vi "setpoint_new(SubVI).vi"(0 "Filed 2":dbl=300.0, 1 "Field":dbl=300.0, 2 "type":T1, 3 "Rate/speed":dbl=10.0, 4 "Mode":i32(ring) items=["Persistent", "Driven"], 5 "输出簇 2":T2={"initialize"=enum."SR830", "6221"={"6221 Resource"="GPIB0::24::INSTR", "Delta status"=FALSE, "电流|RMS(A)"=0.0}, "SR830+6221"={"source"=0, "Current(A)"=0.0, "阻抗(Ohm)"=0.0, "SR830 1"=FALSE, "SR830 2"=FALSE, "SR830 3"=FALSE, "SR830 4"=FALSE, "VISA 1"="", "VISA 2"="", "VISA 3"="", "VISA 4"="", "Reserve 1"=0, "Reserve 2"=-1, "Reserve 3"=-1, "Reserve 4"=-1, "Sensitivity 1"=-1, "Sensitivity 2"=0, "Sensitivity 3"=-1, "Sensitivity 4"=-1, "量程入 1"=0, "量程入 2"=0, "量程入 3"=0, "量程入 4"=0}, "2400"={"2400"=FALSE, "VISA"="", "Output Level (0)"=1e-05, "Compliance  Level (0.1)"=10.0}, "ch"={"ch"=[], "current"=[], "change?"=[], "holding current\nwhen change ch?"=FALSE}, "Instrument"={"325 Resource "="GPIB0::24::INSTR", "Input (0:A) 325"=0, "Heater Output (1:1) 325"=1, "340 Resource"="GPIB0::24::INSTR", "Input (0:A) 340"=0, "Loop (0: 1)"=1, "Input (0:B) 340"=1, "Loop (1: 1)"=2, "340 Status"=refnum, "Instrument Type"=enum."PPMS-Rotate", "quantum design"=refnum, "semaphore 325"=refnum, "TCP master instance"=refnum, "M24C Resource"="GPIB0::24::INSTR", "4G supply"="GPIB0::24::INSTR", "Temp Status 24C"=refnum, "Temp"=refnum, "9T信号"=refnum, "limit"={"Field limit"=0.0, "Field rate limit"=0.0, "Temp limit"=0.0, "Temp low limit"=0.0, "Temp rate limit "=0.0}, "4g supply status"=refnum, "vi路径"="", "in-plane"="", "out-plane"="", "in-plane signal"=FALSE, "out-plane signal"=FALSE, "in plane 信号"=refnum, "pzt volt"=refnum, "Aborting"=refnum, "数据文件"=refnum, "warning"=refnum, "750 visa"="", "750 rotate"="", "335 Status 2"=refnum, "335 Resource "="GPIB0::24::INSTR", "Input (0:A) 335"=0, "Input (0:B) 335"=1, "Heater Output (1:1) 335"=1, "semaphore 340"=refnum, "semaphore 335"=refnum, "325 Status"=refnum, "semaphore 750"=refnum, "750 field status"=refnum}, "2614B"={"2614B chA"=FALSE, "2614B chB"=FALSE, "VISA"=""}, "33522b"={"33522b resource name"="", "零电压"=0.0, "最大电压"=148.0, "间隔"=4.0, "最小电压"=-48.0, "PZT Scan?"=FALSE}, "gating type"=enum."2614(daul)"} {"Instrument"."Loop (1: 1)" items=["1"=1, "2"=2]; "Instrument"."Loop (0: 1)" items=["1"=1, "2"=2]; "Instrument"."Input (0:B) 340" items=["A", "B", "C", "D"]; "Instrument"."Heater Output (1:1) 335" items=["1"=1, "2"=2]; "Instrument"."Input (0:B) 335" items=["A", "B"]; "Instrument"."Input (0:A) 335" items=["A", "B"]; "Instrument"."Heater Output (1:1) 325" items=["1"=1, "2"=2]; "Instrument"."Input (0:A) 325" items=["A", "B"]; "Instrument"."Input (0:A) 340" items=["1"=1, "2"=2]; "SR830+6221"."Sensitivity 4" items=["Auto Gain"=-1, "2 nV/fA"=0, "5 nV/fA"=1, "10 nV/fA"=2, "20 nV/fA"=3, "50 nV/fA"=4, "100 nV/fA"=5, "200 nV/fA"=6, "500 nV/fA"=7, "1 uV/pA"=8, "2 uV/pA"=9, "5 uV/pA"=10, "10 uV/pA"=11, "20 uV/pA"=12, "50 uV/pA"=13, "100 uV/pA"=14, "200 uV/pA"=15, "500 uV/pA"=16, "1 mV/nA"=17, "2 mV/nA"=18, "5 mV/nA"=19, "10 mV/nA"=20, "20 mV/nA"=21, "50 mV/nA"=22, "100 mV/nA"=23, "200 mV/nA"=24, "500 mV/mA"=25, "1 V/uA"=26]; "SR830+6221"."Sensitivity 3" items=["Auto Gain"=-1, "2 nV/fA"=0, "5 nV/fA"=1, "10 nV/fA"=2, "20 nV/fA"=3, "50 nV/fA"=4, "100 nV/fA"=5, "200 nV/fA"=6, "500 nV/fA"=7, "1 uV/pA"=8, "2 uV/pA"=9, "5 uV/pA"=10, "10 uV/pA"=11, "20 uV/pA"=12, "50 uV/pA"=13, "100 uV/pA"=14, "200 uV/pA"=15, "500 uV/pA"=16, "1 mV/nA"=17, "2 mV/nA"=18, "5 mV/nA"=19, "10 mV/nA"=20, "20 mV/nA"=21, "50 mV/nA"=22, "100 mV/nA"=23, "200 mV/nA"=24, "500 mV/mA"=25, "1 V/uA"=26]; "SR830+6221"."Sensitivity 1" items=["Auto Gain"=-1, "2 nV/fA"=0, "5 nV/fA"=1, "10 nV/fA"=2, "20 nV/fA"=3, "50 nV/fA"=4, "100 nV/fA"=5, "200 nV/fA"=6, "500 nV/fA"=7, "1 uV/pA"=8, "2 uV/pA"=9, "5 uV/pA"=10, "10 uV/pA"=11, "20 uV/pA"=12, "50 uV/pA"=13, "100 uV/pA"=14, "200 uV/pA"=15, "500 uV/pA"=16, "1 mV/nA"=17, "2 mV/nA"=18, "5 mV/nA"=19, "10 mV/nA"=20, "20 mV/nA"=21, "50 mV/nA"=22, "100 mV/nA"=23, "200 mV/nA"=24, "500 mV/mA"=25, "1 V/uA"=26]; "SR830+6221"."Sensitivity 2" items=["Auto Gain"=-1, "2 nV/fA"=0, "5 nV/fA"=1, "10 nV/fA"=2, "20 nV/fA"=3, "50 nV/fA"=4, "100 nV/fA"=5, "200 nV/fA"=6, "500 nV/fA"=7, "1 uV/pA"=8, "2 uV/pA"=9, "5 uV/pA"=10, "10 uV/pA"=11, "20 uV/pA"=12, "50 uV/pA"=13, "100 uV/pA"=14, "200 uV/pA"=15, "500 uV/pA"=16, "1 mV/nA"=17, "2 mV/nA"=18, "5 mV/nA"=19, "10 mV/nA"=20, "20 mV/nA"=21, "50 mV/nA"=22, "100 mV/nA"=23, "200 mV/nA"=24, "500 mV/mA"=25, "1 V/uA"=26]; "SR830+6221"."Reserve 4" items=["Auto Gain"=-1, "2 nV/fA"=0, "5 nV/fA"=1, "10 nV/fA"=2, "20 nV/fA"=3, "50 nV/fA"=4, "100 nV/fA"=5, "200 nV/fA"=6, "500 nV/fA"=7, "1 uV/pA"=8, "2 uV/pA"=9, "5 uV/pA"=10, "10 uV/pA"=11, "20 uV/pA"=12, "50 uV/pA"=13, "100 uV/pA"=14, "200 uV/pA"=15, "500 uV/pA"=16, "1 mV/nA"=17, "2 mV/nA"=18, "5 mV/nA"=19, "10 mV/nA"=20, "20 mV/nA"=21, "50 mV/nA"=22, "100 mV/nA"=23, "200 mV/nA"=24, "500 mV/mA"=25, "1 V/uA"=26]; "SR830+6221"."Reserve 3" items=["Auto Reserve"=-1, "High Reserve"=0, "Normal"=1, "Low Noise"=2]; "SR830+6221"."Reserve 2" items=["Auto Reserve"=-1, "High Reserve"=0, "Normal"=1, "Low Noise"=2]; "SR830+6221"."Reserve 1" items=["Auto Reserve"=-1, "High Reserve"=0, "Normal"=1, "Low Noise"=2]; "SR830+6221"."source" items=["SR830 1", "SR830 2", "SR830 3", "SR830 4"]}, 6 "data":refnum<queue>, 7 "Delay":dbl, 9 "steps number":i32, 11 "Approach":i32(ring) items=["FastSettle", "NoOvershoot"], 12 "Source Measure Unit Channel (0: Channel A)":i32(ring) items=["Channel A", "Channel B"], 13 "轴向":enum16{"in plane", "out plane"}(ring)) -> (8 "错误输出":errorcluster, 15 "输出簇":T2={"initialize"=enum."SR830", "6221"={"6221 Resource"="GPIB0::24::INSTR", "Delta status"=FALSE, "电流|RMS(A)"=0.0}, "SR830+6221"={"source"=0, "Current(A)"=0.0, "阻抗(Ohm)"=0.0, "SR830 1"=FALSE, "SR830 2"=FALSE, "SR830 3"=FALSE, "SR830 4"=FALSE, "VISA 1"="", "VISA 2"="", "VISA 3"="", "VISA 4"="", "Reserve 1"=0, "Reserve 2"=-1, "Reserve 3"=-1, "Reserve 4"=-1, "Sensitivity 1"=-1, "Sensitivity 2"=0, "Sensitivity 3"=-1, "Sensitivity 4"=-1, "量程入 1"=0, "量程入 2"=0, "量程入 3"=0, "量程入 4"=0}, "2400"={"2400"=FALSE, "VISA"="", "Output Level (0)"=1e-05, "Compliance  Level (0.1)"=10.0}, "ch"={"ch"=[], "current"=[], "change?"=[], "holding current\nwhen change ch?"=FALSE}, "Instrument"={"325 Resource "="GPIB0::24::INSTR", "Input (0:A) 325"=0, "Heater Output (1:1) 325"=1, "340 Resource"="GPIB0::24::INSTR", "Input (0:A) 340"=0, "Loop (0: 1)"=1, "Input (0:B) 340"=1, "Loop (1: 1)"=2, "340 Status"=refnum, "Instrument Type"=enum."PPMS-Rotate", "quantum design"=refnum, "semaphore 325"=refnum, "TCP master instance"=refnum, "M24C Resource"="GPIB0::24::INSTR", "4G supply"="GPIB0::24::INSTR", "Temp Status 24C"=refnum, "Temp"=refnum, "9T信号"=refnum, "limit"={"Field limit"=0.0, "Field rate limit"=0.0, "Temp limit"=0.0, "Temp low limit"=0.0, "Temp rate limit "=0.0}, "4g supply status"=refnum, "vi路径"="", "in-plane"="", "out-plane"="", "in-plane signal"=FALSE, "out-plane signal"=FALSE, "in plane 信号"=refnum, "pzt volt"=refnum, "Aborting"=refnum, "数据文件"=refnum, "warning"=refnum, "750 visa"="", "750 rotate"="", "335 Status 2"=refnum, "335 Resource "="GPIB0::24::INSTR", "Input (0:A) 335"=0, "Input (0:B) 335"=1, "Heater Output (1:1) 335"=1, "semaphore 340"=refnum, "semaphore 335"=refnum, "325 Status"=refnum, "semaphore 750"=refnum, "750 field status"=refnum}, "2614B"={"2614B chA"=FALSE, "2614B chB"=FALSE, "VISA"=""}, "33522b"={"33522b resource name"="", "零电压"=0.0, "最大电压"=148.0, "间隔"=4.0, "最小电压"=-48.0, "PZT Scan?"=FALSE}, "gating type"=enum."2614(daul)"} {"Instrument"."Loop (1: 1)" items=["1"=1, "2"=2]; "Instrument"."Loop (0: 1)" items=["1"=1, "2"=2]; "Instrument"."Input (0:B) 340" items=["A", "B", "C", "D"]; "Instrument"."Heater Output (1:1) 335" items=["1"=1, "2"=2]; "Instrument"."Input (0:B) 335" items=["A", "B"]; "Instrument"."Input (0:A) 335" items=["A", "B"]; "Instrument"."Heater Output (1:1) 325" items=["1"=1, "2"=2]; "Instrument"."Input (0:A) 325" items=["A", "B"]; "Instrument"."Input (0:A) 340" items=["1"=1, "2"=2]; "SR830+6221"."Sensitivity 4" items=["Auto Gain"=-1, "2 nV/fA"=0, "5 nV/fA"=1, "10 nV/fA"=2, "20 nV/fA"=3, "50 nV/fA"=4, "100 nV/fA"=5, "200 nV/fA"=6, "500 nV/fA"=7, "1 uV/pA"=8, "2 uV/pA"=9, "5 uV/pA"=10, "10 uV/pA"=11, "20 uV/pA"=12, "50 uV/pA"=13, "100 uV/pA"=14, "200 uV/pA"=15, "500 uV/pA"=16, "1 mV/nA"=17, "2 mV/nA"=18, "5 mV/nA"=19, "10 mV/nA"=20, "20 mV/nA"=21, "50 mV/nA"=22, "100 mV/nA"=23, "200 mV/nA"=24, "500 mV/mA"=25, "1 V/uA"=26]; "SR830+6221"."Sensitivity 3" items=["Auto Gain"=-1, "2 nV/fA"=0, "5 nV/fA"=1, "10 nV/fA"=2, "20 nV/fA"=3, "50 nV/fA"=4, "100 nV/fA"=5, "200 nV/fA"=6, "500 nV/fA"=7, "1 uV/pA"=8, "2 uV/pA"=9, "5 uV/pA"=10, "10 uV/pA"=11, "20 uV/pA"=12, "50 uV/pA"=13, "100 uV/pA"=14, "200 uV/pA"=15, "500 uV/pA"=16, "1 mV/nA"=17, "2 mV/nA"=18, "5 mV/nA"=19, "10 mV/nA"=20, "20 mV/nA"=21, "50 mV/nA"=22, "100 mV/nA"=23, "200 mV/nA"=24, "500 mV/mA"=25, "1 V/uA"=26]; "SR830+6221"."Sensitivity 1" items=["Auto Gain"=-1, "2 nV/fA"=0, "5 nV/fA"=1, "10 nV/fA"=2, "20 nV/fA"=3, "50 nV/fA"=4, "100 nV/fA"=5, "200 nV/fA"=6, "500 nV/fA"=7, "1 uV/pA"=8, "2 uV/pA"=9, "5 uV/pA"=10, "10 uV/pA"=11, "20 uV/pA"=12, "50 uV/pA"=13, "100 uV/pA"=14, "200 uV/pA"=15, "500 uV/pA"=16, "1 mV/nA"=17, "2 mV/nA"=18, "5 mV/nA"=19, "10 mV/nA"=20, "20 mV/nA"=21, "50 mV/nA"=22, "100 mV/nA"=23, "200 mV/nA"=24, "500 mV/mA"=25, "1 V/uA"=26]; "SR830+6221"."Sensitivity 2" items=["Auto Gain"=-1, "2 nV/fA"=0, "5 nV/fA"=1, "10 nV/fA"=2, "20 nV/fA"=3, "50 nV/fA"=4, "100 nV/fA"=5, "200 nV/fA"=6, "500 nV/fA"=7, "1 uV/pA"=8, "2 uV/pA"=9, "5 uV/pA"=10, "10 uV/pA"=11, "20 uV/pA"=12, "50 uV/pA"=13, "100 uV/pA"=14, "200 uV/pA"=15, "500 uV/pA"=16, "1 mV/nA"=17, "2 mV/nA"=18, "5 mV/nA"=19, "10 mV/nA"=20, "20 mV/nA"=21, "50 mV/nA"=22, "100 mV/nA"=23, "200 mV/nA"=24, "500 mV/mA"=25, "1 V/uA"=26]; "SR830+6221"."Reserve 4" items=["Auto Gain"=-1, "2 nV/fA"=0, "5 nV/fA"=1, "10 nV/fA"=2, "20 nV/fA"=3, "50 nV/fA"=4, "100 nV/fA"=5, "200 nV/fA"=6, "500 nV/fA"=7, "1 uV/pA"=8, "2 uV/pA"=9, "5 uV/pA"=10, "10 uV/pA"=11, "20 uV/pA"=12, "50 uV/pA"=13, "100 uV/pA"=14, "200 uV/pA"=15, "500 uV/pA"=16, "1 mV/nA"=17, "2 mV/nA"=18, "5 mV/nA"=19, "10 mV/nA"=20, "20 mV/nA"=21, "50 mV/nA"=22, "100 mV/nA"=23, "200 mV/nA"=24, "500 mV/mA"=25, "1 V/uA"=26]; "SR830+6221"."Reserve 3" items=["Auto Reserve"=-1, "High Reserve"=0, "Normal"=1, "Low Noise"=2]; "SR830+6221"."Reserve 2" items=["Auto Reserve"=-1, "High Reserve"=0, "Normal"=1, "Low Noise"=2]; "SR830+6221"."Reserve 1" items=["Auto Reserve"=-1, "High Reserve"=0, "Normal"=1, "Low Noise"=2]; "SR830+6221"."source" items=["SR830 1", "SR830 2", "SR830 3", "SR830 4"]})   [LabVIEW 2019, in "Scan.lvlib"]
uses:
  Scan.lvlib
  ctl/config.ctl
  <vilib>/NI/Modbus Library/API/Master/Modbus Master.lvclass
  ctl/initialize.ctl
  ctl/Instrument.ctl
  ctl/335 state.ctl
  ctl/Instrument Type.ctl
  lib/QDInstrument.dll
  ctl/limit.ctl
  ctl/9T mag field stauts.ctl
  ctl/warning.ctl
  ctl/Gating type.ctl
  ctl/set type.ctl
  SubVI.lvlib
  nematic.lvlib
  User lib.lvlib
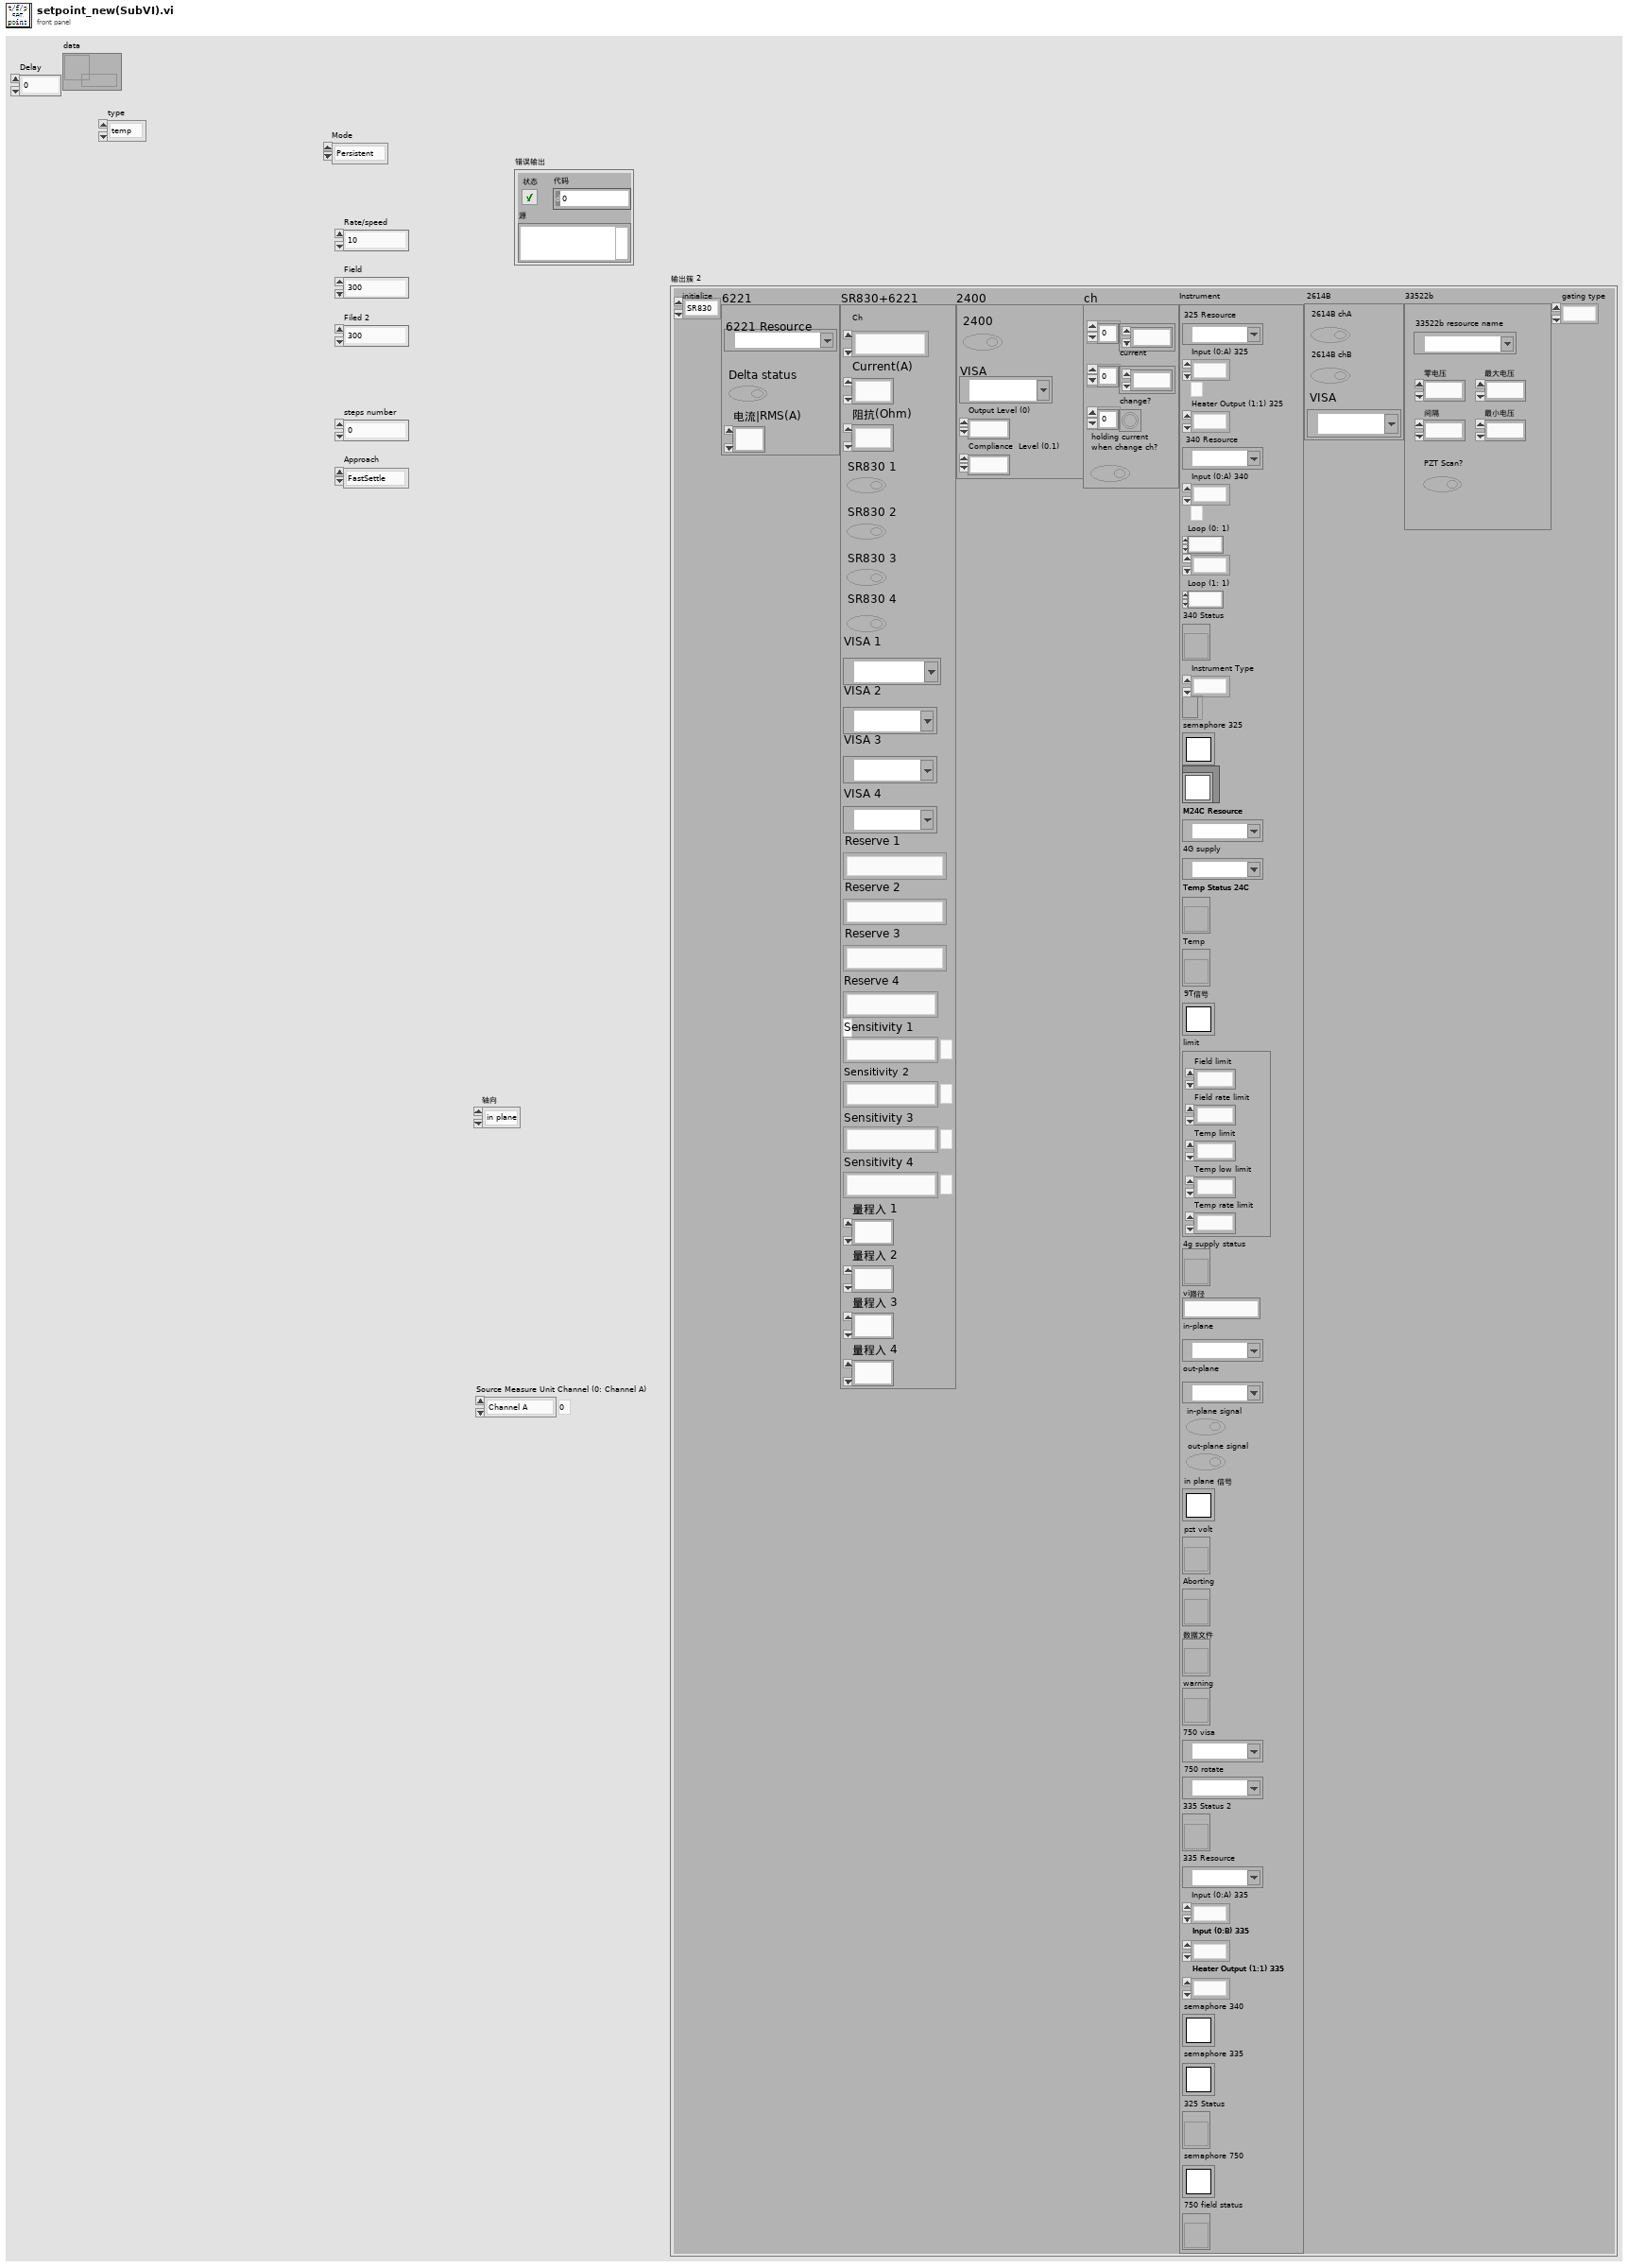
[diagram p1: front panel]
types:
  T1 = typedef "set type.ctl" = enum16{"temp", "field", "position", "gating", "current"}
  T2 = typedef "config.ctl" = cluster{"initialize":T3, "6221":cluster{"6221 Resource":refnum<visa-resource-name>, "Delta status":bool, "电流|RMS(A)":dbl}, "SR830+6221":cluster{"source":u16, "Current(A)":dbl, "阻抗(Ohm)":dbl, "SR830 1":bool, "SR830 2":bool, "SR830 3":bool, "SR830 4":bool, "VISA 1":refnum<visa-resource-name>, "VISA 2":refnum<visa-resource-name>, "VISA 3":refnum<visa-resource-name>, "VISA 4":refnum<visa-resource-name>, "Reserve 1":i16, "Reserve 2":i16, "Reserve 3":i16, "Reserve 4":i16, "Sensitivity 1":i16, "Sensitivity 2":i16, "Sensitivity 3":i16, "Sensitivity 4":i16, "量程入 1":i32, "量程入 2":i32, "量程入 3":i32, "量程入 4":i32}, "2400":cluster{"2400":bool, "VISA":refnum<visa-resource-name>, "Output Level (0)":dbl, "Compliance  Level (0.1)":dbl}, "ch":cluster{"ch":i32[], "current":dbl[], "change?":bool[], "holding current\nwhen change ch?":bool}, "Instrument":T4, "2614B":cluster{"2614B chA":bool, "2614B chB":bool, "VISA":refnum<visa-resource-name>}, "33522b":cluster{"33522b resource name":refnum<visa-resource-name>, "零电压":dbl, "最大电压":dbl, "间隔":dbl, "最小电压":dbl, "PZT Scan?":bool}, "gating type":T8}
  T3 = typedef "initialize.ctl" = enum16{"SR830", "keithley6221-SR830", "Delta", "Delta-tunnelling", "keithley6221-2182-DC", "PZT"}
  T4 = typedef "Instrument.ctl" = cluster{"325 Resource ":refnum<visa-resource-name>, "Input (0:A) 325":u16, "Heater Output (1:1) 325":u16, "340 Resource":refnum<visa-resource-name>, "Input (0:A) 340":u16, "Loop (0: 1)":u16, "Input (0:B) 340":u16, "Loop (1: 1)":u16, "340 Status":refnum<vi>, "Instrument Type":T5, "quantum design":refnum<k24>, "semaphore 325":T6, "TCP master instance":refnum<class "Modbus Master.lvclass">, "M24C Resource":refnum<visa-resource-name>, "4G supply":refnum<visa-resource-name>, "Temp Status 24C":refnum<vi>, "Temp":refnum<vi>, "9T信号":T6, "limit":T7, "4g supply status":refnum<vi>, "vi路径":string, "in-plane":refnum<visa-resource-name>, "out-plane":refnum<visa-resource-name>, "in-plane signal":bool, "out-plane signal":bool, "in plane 信号":T6, "pzt volt":refnum<vi>, "Aborting":refnum<vi>, "数据文件":refnum<vi>, "warning":refnum<vi>, "750 visa":refnum<visa-resource-name>, "750 rotate":refnum<visa-resource-name>, "335 Status 2":refnum<vi>, "335 Resource ":refnum<visa-resource-name>, "Input (0:A) 335":u16, "Input (0:B) 335":u16, "Heater Output (1:1) 335":u16, "semaphore 340":T6, "semaphore 335":T6, "325 Status":refnum<vi>, "semaphore 750":T6, "750 field status":refnum<vi>}
  T5 = typedef "Instrument Type.ctl" = enum16{"PPMS", "VersaLab", "DynaCool", "SVSM", "PPMS-Rotate", "Lakeshore335", "lengtou2", "9T mag", "9T cmag rotate", "test"}
  T6 = typedef "Semaphore RefNum" = refnum<k1>
  T7 = typedef "limit.ctl" = cluster{"Field limit":dbl, "Field rate limit":dbl, "Temp limit":dbl, "Temp low limit":dbl, "Temp rate limit ":dbl}
  T8 = typedef "Gating type.ctl" = enum32{"null", "2614(daul)", "2400"}
  T9 = cluster{"temp":bool, "field":bool, "position":bool, "charmbe":bool}
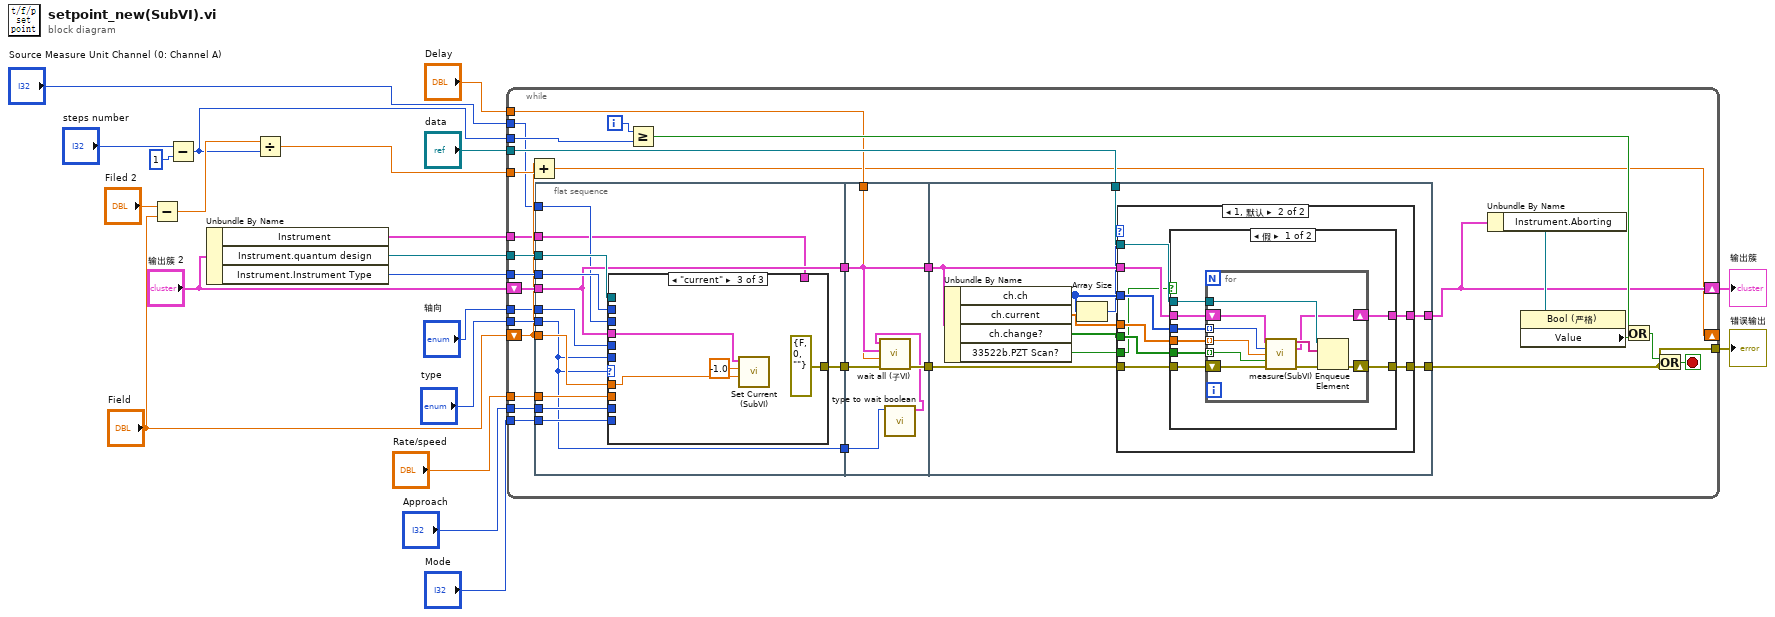
[diagram p0: block diagram]
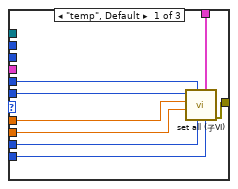
[diagram p2: hidden frame]
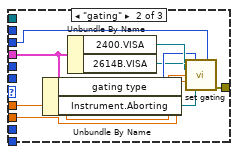
[diagram p3: hidden frame]
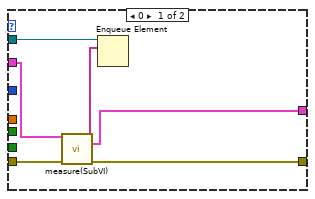
[diagram p4: hidden frame]
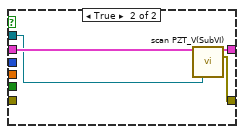
[diagram p5: hidden frame]
diagram:
  n1 = Subtract(x="Filed 2", y="Field") -> (x-y=w21:dbl)
  n2 = Subtract(x="steps number", y=1) -> (x-y=w13:i32)
  n3 = Unbundle By Name("输出簇 2") -> ("Instrument"=w1:T4, "Instrument.quantum design"=w10:refnum<k24>, "Instrument.Instrument Type"=w9:T5)
  n4 = Divide(x=w21, y=w13) -> (x/y=w7:dbl)
  n5 = while {
    tunnel: w13 -> [w48]
    tunnel: "data" -> [w50]
    tunnel: "Mode" -> [w46]
    tunnel: "Approach" -> [w45]
    tunnel: "Rate/speed" -> [w44]
    tunnel: w10 -> [w43]
    tunnel: [w37] -> w16
    tunnel: "Delay" -> [w38]
    tunnel: "type" -> [w36]
    tunnel: w9 -> [w35]
    shift-right: [w26] -> _
    shift-left: "Field" -> [w27]
    tunnel: w7 -> [w28]
    shift-right: [w31] -> w6
    shift-left: "输出簇 2" -> [w29]
    tunnel: "Source Measure Unit Channel (0: Channel A)" -> [w25]
    tunnel: "轴向" -> [w24]
    tunnel: w1 -> [w22]
    i -> [w47]
    stop <- w41 stop-if-true
    n6 = Add(x=w28, y=w27) -> (x+y=w26:dbl)
    n7 = flat-sequence {
      tunnel: w46 -> [w62]
      tunnel: w45 -> [w61]
      tunnel: w44 -> [w60]
      tunnel: w43 -> [w59]
      tunnel: [w58] -> w40
      tunnel: w36 -> [w52]
      tunnel: w35 -> [w57]
      tunnel: w27 -> [w55]
      tunnel: w29 -> [w56]
      tunnel: [w56] -> w30
      tunnel: w25 -> [w54]
      tunnel: w24 -> [w53]
      tunnel: [w52] -> w23
      tunnel: w22 -> [w51]
      tunnel: w40 -> [w87]
      tunnel: [w86] -> w39
      tunnel: w38 -> [w88]
      tunnel: [w89] -> w34
      tunnel: w30 -> [w89]
      tunnel: w23 -> [w85]
      tunnel: [w94] -> w37
      tunnel: w39 -> [w93]
      tunnel: w50 -> [w98]
      tunnel: w34 -> [w99]
      tunnel: [w95] -> w31
      frame #0 {
        n8 = case shown="\"current\"" w52 {
          tunnel: w62 -> [w65 _ _]
          tunnel: w61 -> [w66 _ _]
          tunnel: w60 -> [w69 w76 _]
          tunnel: w59 -> [_ _ _]
          tunnel: [w68 w72 errorcluster {"status"=FALSE, "code"=0, "source"=""} ("error out")] -> w58
          tunnel: w52 -> [w70 _ _]
          tunnel: w57 -> [_ _ _]
          tunnel: w56 -> [_ w79 w83]
          tunnel: w55 -> [w64 w77 w82]
          tunnel: w54 -> [_ w74 _]
          tunnel: w53 -> [w67 _ _]
          tunnel: w51 -> [w63 _ _]
          frame "temp", Default {
            n9 = call "set all (子VI).vi"("Mode(ppms,mpms磁)"=w65, "Instrument"=w63, "Approach(ppms, mpms)"=w66, "轴向(转角)"=w67, "Rate/speed"=w69, "Target"=w64, "类型"=w70) -> ("error out"=w68:errorcluster)  [unwired: 4 in]
          }
          frame "gating" {
            n10 = Unbundle By Name(w79) -> ("gating type"=w75:T8, "Instrument.Aborting"=w73:refnum<vi>)
            n11 = Unbundle By Name(w79) -> ("2400.VISA"=w78:refnum<visa-resource-name>, "2614B.VISA"=w71:refnum<visa-resource-name>)
            n12 = call "set gating.vi"("2400 VISA"=w78, "gating type"=w75, "Source Measure Unit Channel (0: Channel A)"=w74, "2614 VISA"=w71, "Voltage Level"=w77, "RATE(mV/s)"=w76, "abort"=w73) -> ("error out"=w72:errorcluster)  [unwired: 7 in, 1 out]
          }
          frame "current" {
            n13 = call "Set Current (SubVI).vi"("current(A)"=w82, "freq"=-1.0, "config"=w83) -> ()  [unwired: 8 in, 1 out]
          }
        }
      }
      frame #1 {
        n14 = call "type to wait boolean.vi"("类型"=w85) -> ("簇"=w84:T9)  [unwired: 10 in]
        n15 = call "wait all (子VI).vi"("错误输入（无错误）"=w87, "delay"=w88, "输出簇输入"=w89, "Boolean"=w84) -> ("错误输出"=w86:errorcluster)  [unwired: 7 in]
      }
      frame #2 {
        n16 = Unbundle By Name(w99) -> ("ch.ch"=w92:i32[], "ch.current"=w97:dbl[], "ch.change?"=w96:bool[], "33522b.PZT Scan?"=w90:bool)
        n17 = Array Size(array=w92) -> (size(s)=w91:i32)
        n18 = case shown="1, 默认" w91 {
          tunnel: w99 -> [w105 w114]
          tunnel: w92 -> [_ w113]
          tunnel: w97 -> [_ w112]
          tunnel: w96 -> [_ w111]
          tunnel: w98 -> [w100 w110]
          tunnel: w93 -> [w104 w109]
          tunnel: [w103 w108] -> w94
          tunnel: [w102 w107] -> w95
          tunnel: w90 -> [_ w106]
          frame 0 {
            n19 = call "measure(SubVI).vi"("config in"=w105, "error in (no error)"=w104) -> ("data"=w101:string[], "config out"=w102:T2, "error out"=w103:errorcluster)  [unwired: 11 in]
            n20 = Enqueue Element(queue=w100, element=w101) -> ()  [unwired: 2 in, 3 out]
          }
          frame 1, Default {
            n21 = case shown="假" w106 {
              tunnel: w114 -> [w122 w136]
              tunnel: w113 -> [w121 _]
              tunnel: w112 -> [w120 _]
              tunnel: w111 -> [w119 _]
              tunnel: w110 -> [w118 w135]
              tunnel: w109 -> [w117 _]
              tunnel: [w116 w133] -> w108
              tunnel: [w115 w134] -> w107
              frame False {
                n22 = for {
                  tunnel: w121 -> [w130] mode=indexing
                  tunnel: w119 -> [w128] mode=indexing
                  tunnel: w120 -> [w129] mode=indexing
                  tunnel: w118 -> [w132]
                  shift-right: [w126] -> w115
                  shift-left: w122 -> [w131]
                  shift-right: [w123] -> w116
                  shift-left: w117 -> [w125]
                  n23 = call "measure(SubVI).vi"("config in"=w131, "ch"=w130, "current"=w129, "change?"=w128, "error in (no error)"=w125) -> ("data"=w127:string[], "config out"=w126:T2, "error out"=w124:errorcluster)  [unwired: 8 in]
                  n24 = Enqueue Element(queue=w132, element=w127, error in (no error)=w124) -> (error out=w123:errorcluster)  [unwired: 1 in, 2 out]
                }
              }
              frame True {
                n25 = call "scan PZT_V(SubVI).vi"("config"=w136, "data"=w135) -> ("输出簇"=w134:T2, "错误输出"=w133:errorcluster)  [unwired: 12 in]
              }
            }
          }
        }
      }
    }
    n26 = Greater Or Equal?(x=w47, y=w48) -> (x >= y?=w49:bool)
    n27 = Unbundle By Name(w31) -> ("Instrument.Aborting"=w33:refnum<vi>)
    n28 = property class="Bool (严格)"(reference=w33) -> ("Value"=w32:bool)  [unwired: 1 in, 2 out]
    n29 = Or(x=w49, y=w32) -> (x .or. y?=w42:bool)
    n30 = Or(x=w42, y=w37) -> (x .or. y?=w41:bool)
  }
  "错误输出" <- w16
  "输出簇" <- w6
